vi "Update Fan Status.vi"(8 "error in (no error)":cluster{"状态":bool, "代码":i32, "源":string} caption="错误输入（无错误）", 9 "风扇B":T1, 10 "风扇A":T1, 11 "蒸发冷却器的控制器输入":refnum<class "Evaporative Cooler Controller.lvclass">) -> (0 "error out":cluster{"状态":bool, "代码":i32, "源":string} caption="错误输出", 3 "蒸发冷却器的控制器输出":refnum<class "Evaporative Cooler Controller.lvclass">)   [LabVIEW 2015, in "Evaporative Cooler Controller.lvlib" / "Evaporative Cooler Controller.lvclass"]
doc: "子类中必须对该方法进行重写以显示风扇的新状态或更新记录文件。"
uses:
  Evaporative Cooler Controller.lvclass
  Dual Fan/Dual Fan/Fan Info.ctl
  Dual Fan/Dual Fan/Dual Fan.lvclass
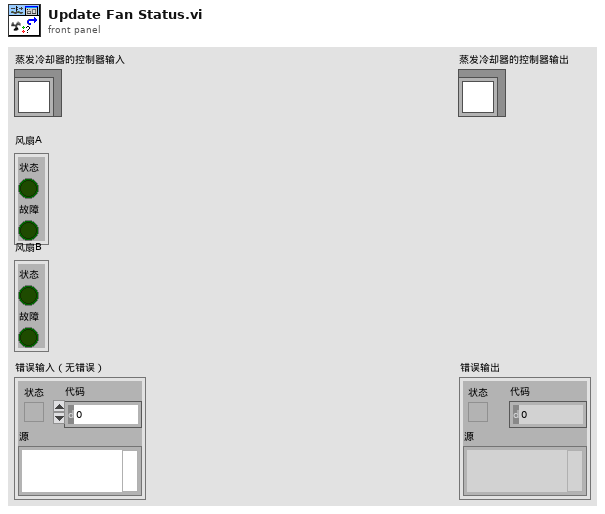
[diagram p1: front panel]
types:
  T1 = typedef "Dual Fan.lvlib/Dual Fan.lvclass/Fan Info.ctl" = cluster{"状态":bool, "故障":bool}
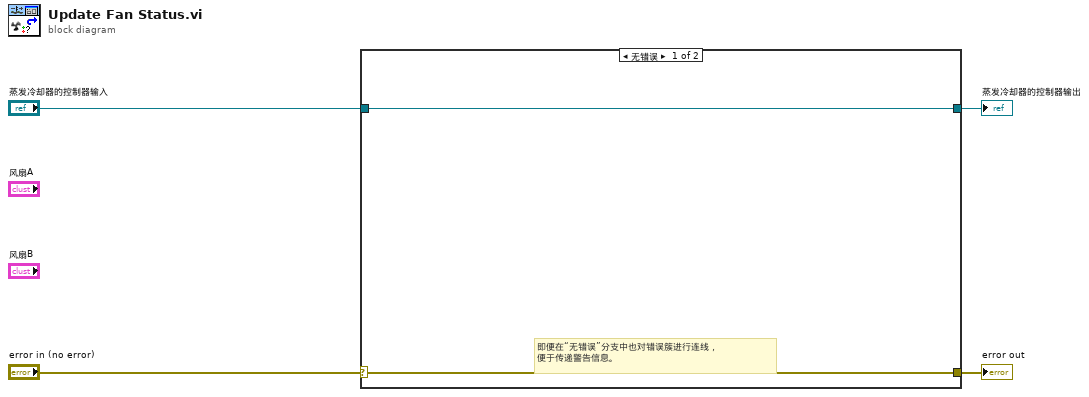
[diagram p0: block diagram]
diagram:
  n1 = case shown="无错误" "error in (no error)" {
    selector: "error in (no error)" -> [w5 w8]
    tunnel: [w5 w8] -> w3
    tunnel: [w6 w7] -> w1
    tunnel: "蒸发冷却器的控制器输入" -> [w6 w7]
    frame No Error {
      # "即便在“无错误”分支中也对错误簇进行连线，\n便于传递警告信息。"
    }
    frame Error {
    }
  }
  "error out" <- w3
  "蒸发冷却器的控制器输出" <- w1
